vi "IntSignal (SubVI).vi"(8 "error in (no error)":errorcluster, 9 "channel":u16, 10 "integration":i32, 11 "Application in":refnum<vi>) -> (0 "error out":errorcluster, 2 "Signal value":sgl, 3 "Application out":refnum<vi>)   [LabVIEW 2014]
uses:
  <userlib>/Nanonis Prog Interface V5/Nanonis Prog Interface.lvlib
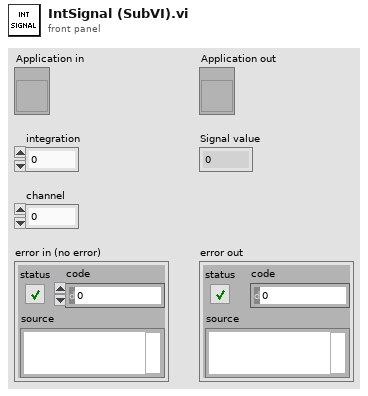
[diagram p1: front panel]
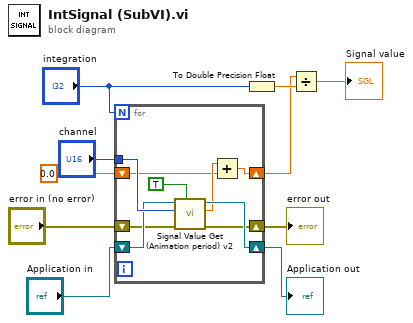
[diagram p0: block diagram]
diagram:
  n1 = for {
    N: "integration" -> [_]
    tunnel: "channel" -> [w19]
    shift-right: [w16] -> w9
    shift-left: "Application in" -> [w18]
    shift-right: [w15] -> w10
    shift-left: "error in (no error)" -> [w17]
    shift-right: [w11] -> w2
    shift-left: sgl 0.0 -> [w12]
    n2 = call <userlib>:"Signal Value Get (Animation period) v2.vi"("Wait for newest data (F=False)"=TRUE, "error in (no error)"=w17, "Signal index (0-79)"=w19, "Application ref in"=w18) -> ("error out"=w15:errorcluster, "Signal value"=w13:sgl, "Application ref out"=w16:refnum<vi>)  [unwired: 4 in]
    n3 = Add(x=w13, y=w12) -> (x+y=w11:sgl)
  }
  "error out" <- w10
  "Application out" <- w9
  n4 = To Double Precision Float(number="integration") -> (double precision float=w3:dbl)
  n5 = Divide(x=w2, y=w3) -> (x/y=→"Signal value":dbl)
